vi "double_arr_to_bool_arr (sub-vi).vi"(5 "double array":dbl[](array[numeric])) -> (2 "bool array":bool[](array[boolean]))   [LabVIEW 2021]
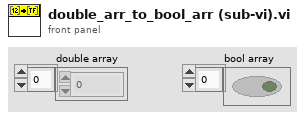
[diagram p1: front panel]
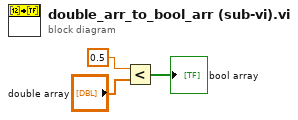
[diagram p0: block diagram]
diagram:
  n1 = Less?(x=0.5, y="double array") -> (x < y?=→"bool array":bool[])
